vi "Dapper Testbed.vi"() -> ()   [LabVIEW 2024]
uses:
  AlbumMap/AlbumMap.lvclass
  Album/Album.lvclass
  b1d846c9-6986-4a9f-951f-cc365dbfe813.vi
  ORM_API/ORM_API.lvlib
  dcba7a19-1003-47d0-b589-a3f07eba521e.vi
  <vilib>/Viviota/shared/ORM_DBC_Mssql.lvlibp/SQL Connect.vi
  <vilib>/Viviota/shared/ORM_DBC_Mssql.lvlibp/DBC.lvclass
panel:
  out "Value":variant
  out "Array":cluster{"Primary Key":i64, "Title":string}[](array[cluster])
  in  "cycles":i32=10
  out "Average Time Per Cycle":dbl
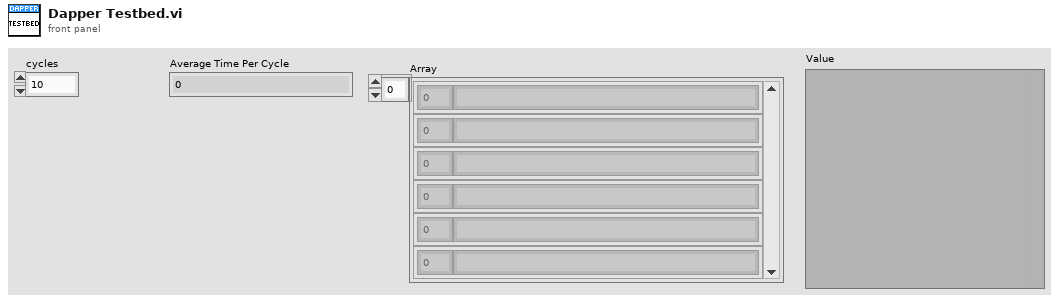
[diagram p1: front panel]
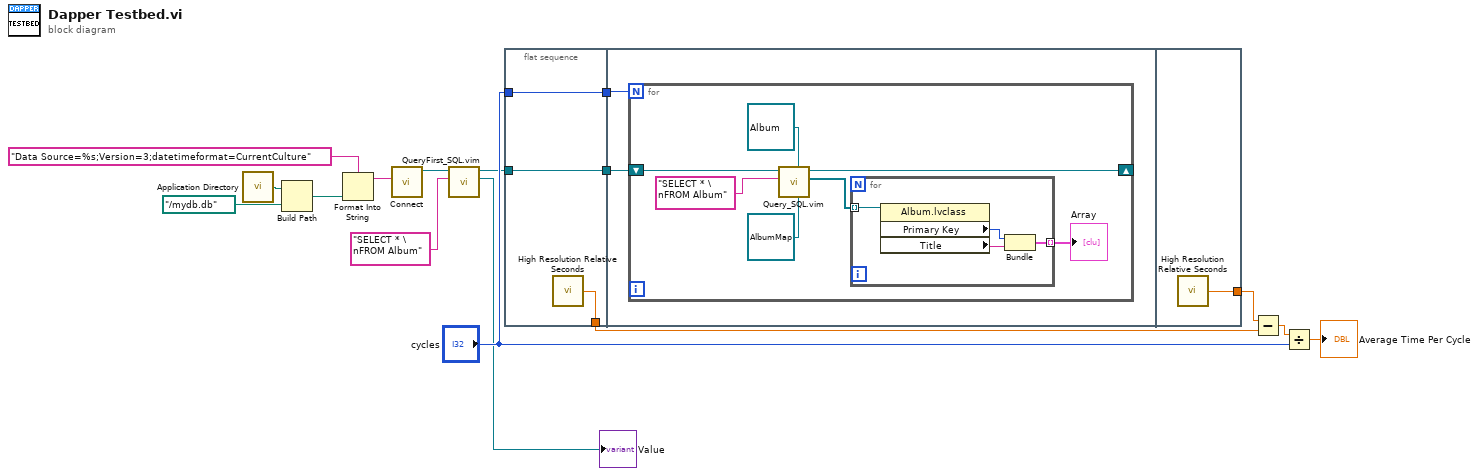
[diagram p0: block diagram]
diagram:
  n1 = call <vilib>:"Application Directory.vi"() -> ("Application Directory"=w7:path)
  n2 = Build Path(base path=w7, name or relative path=path "../mydb.db" ("file out")) -> (appended path=w6:path)
  n3 = Format Into String(format string="Data Source=%s;Version=3;datetimeformat=CurrentCulture" ("connectionStringName"), w6) -> (resulting string=w1:string)  [unwired: 2 in, 1 out]
  n4 = call-poly "Connect.vi"("Connection String"=w1) -> ("SQL Mapper"=w2:refnum<class "SqlMapper.lvclass">)  [unwired: 9 in, 1 out]
  n5 = call "QueryFirst_SQL.vim"("sql"="SELECT * \nFROM Album", "SqlMapper in"=w2) -> ("Value"=→"Value":refnum<class>, "SqlMapper out"=w5:refnum<class "SqlMapper.lvclass">)  [unwired: 7 in, 1 out]
  n6 = flat-sequence {
    tunnel: "cycles" -> [w19]
    tunnel: [w19] -> w16
    tunnel: [w18] -> w14
    tunnel: w5 -> [w17]
    tunnel: [w17] -> w13
    tunnel: w16 -> [w21]
    tunnel: w13 -> [w20]
    tunnel: [w33] -> w15
    frame #0 {
      n7 = call <vilib>:"High Resolution Relative Seconds.vi"() -> ("relative seconds"=w18:dbl)
    }
    frame #1 {
      n8 = for {
        N: w21 -> [_]
        shift-right: [w24] -> _
        shift-left: w20 -> [w27]
        n9 = call "Query_SQL.vim"("TypeMap"=refnum<class "AlbumMap.lvclass"> refnum ("AlbumMap.lvclass"), "type"=refnum<class "Album.lvclass"> refnum ("Album.lvclass"), "sql"="SELECT * \nFROM Album", "SqlMapper in"=w27) -> ("Results"=w23:refnum<class "Album.lvclass">[], "SqlMapper out"=w24:refnum<class "SqlMapper.lvclass">)  [unwired: 5 in, 1 out]
        n10 = for {
          tunnel: w23 -> [w32] mode=indexing
          tunnel: [w29] -> w28 mode=indexing
          n11 = property class="Album.lvclass"(reference=w32) -> ("Primary Key"=w31:i64, "Title"=w30:string)  [unwired: 1 in, 2 out]
          n12 = Bundle("Primary Key"=w31, "Title"=w30) -> (w29:cluster{"Primary Key":i64, "Title":string})  [unwired: 1 in]
        }
        "Array" <- w28
      }
    }
    frame #2 {
      n13 = call <vilib>:"High Resolution Relative Seconds.vi"() -> ("relative seconds"=w33:dbl)
    }
  }
  n14 = Subtract(x=w15, y=w14) -> (x-y=w12:dbl)
  n15 = Divide(x=w12, y="cycles") -> (x/y=→"Average Time Per Cycle":dbl)
